vi "EV3_InitializationRoutine.vi"(8 "error in (no error)":errorcluster, 9 "Console In":string, 11 "Python in":cluster{"Python":refnum<k35>, "py file":path}) -> (0 "error out":errorcluster, 1 "Console Out":string="\n\n", 3 "Python out":cluster{"Python":refnum<k35>, "py file":path})   [LabVIEW 2020]
uses:
  <vilib>/Utility/error.llb/DialogType.ctl
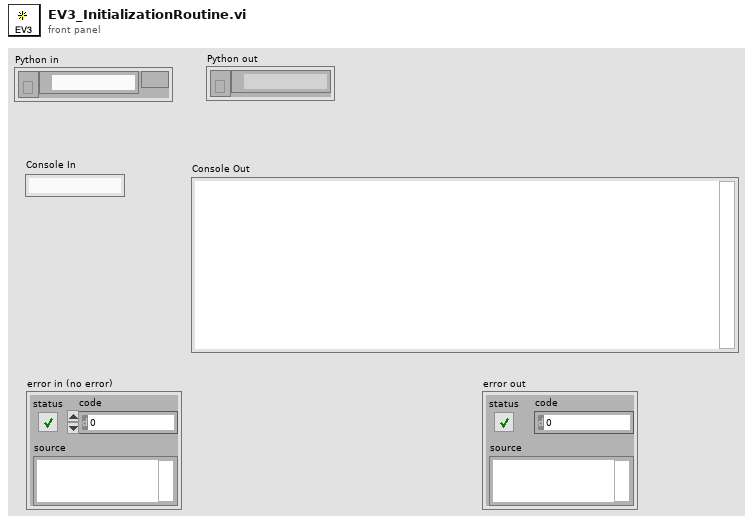
[diagram p1: front panel]
types:
  T1 = typedef "DialogType.ctl" = u16
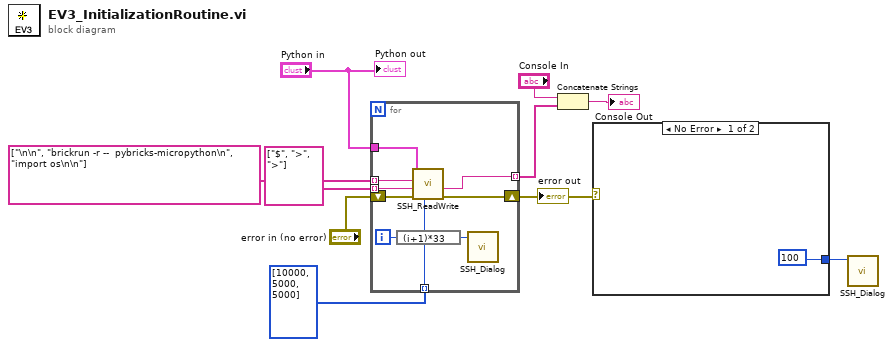
[diagram p0: block diagram]
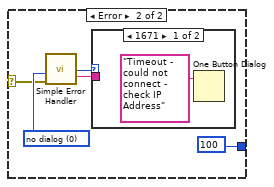
[diagram p2: hidden frame]
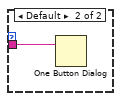
[diagram p3: hidden frame]
diagram:
  n1 = for {
    tunnel: "Python in" -> [w19]
    shift-right: [w17] -> w6
    shift-left: "error in (no error)" -> [w18]
    tunnel: string[] ["\n\n", "brickrun -r --  pybricks-micropython\n", "import os\n\n"] -> [w16] mode=indexing
    tunnel: string[] ["$", ">", ">"] -> [w15] mode=indexing
    tunnel: u32[] [10000, 5000, 5000] -> [w14] mode=indexing
    tunnel: [w13] -> w3 mode=indexing
    i -> [w12]
    n2 = expression code="(i+1)*33"(w12) -> (w11:i32)
    n3 = call "SSH_ReadWrite.vi"("Timeout (ms)"=w14, "error in (no error)"=w18, "Wait for"=w15, "To Send"=w16, "Python in"=w19) -> ("error out"=w17:errorcluster, "Console"=w13:string)  [unwired: 5 in]
    n4 = call "SSH_Dialog.vi"("Slide"=w11) -> ()  [unwired: 11 in]
  }
  "error out" <- w6
  n5 = Concatenate Strings("Console In", w3) -> (→"Console Out":string)
  n6 = case shown="No Error" w6 {
    selector: w6 -> [_ w24]
    tunnel: [u8 100 ("Slide") u8 100 ("Slide")] -> w5
    frame No Error {
    }
    frame Error {
      w25 = T1 0 items=["no dialog", "OK message", "continue or stop message", "OK message + warnings", "continue/stop + warnings"] ("type of dialog (OK msg:1)")
      n7 = call <vilib>:"Simple Error Handler.vi"("type of dialog (OK msg:1)"=w25, "error in (no error)"=w24) -> ("code out"=w21:i32, "message"=w23:string)  [unwired: 3 in, 3 out]
      n8 = case shown="1671" w21 {
        tunnel: w23 -> [_ w27]
        frame 1671 {
          n9 = One Button Dialog(message="Timeout - could not connect - check IP Address") -> ()  [unwired: 1 in, 1 out]
        }
        frame Default {
          n10 = One Button Dialog(message=w27) -> ()  [unwired: 1 in, 1 out]
        }
      }
    }
  }
  n11 = call "SSH_Dialog.vi"("Slide"=w5) -> ()  [unwired: 11 in]
  "Python out" <- "Python in"
